vi "SQL_Delete.vi"(7 "表名":string, 8 "error in (no error)":errorcluster, 9 "值":string, 10 "列名":string, 11 "connection reference":T1) -> (0 "error out":errorcluster, 3 "connection reference 2":T1)   [LabVIEW 2018]
uses:
  <vilib>/addons/database/Connection.llb/Conn ObjectReference.ctl
  <vilib>/addons/database/Connection.llb/Conn Execute.vi
  <vilib>/addons/database/Recordset.llb/Rec Destroy - Connection.vi
  <vilib>/addons/database/NI_Database_API.lvlib
panel:
  # "语法："
  # "DELETE FROM 表名称 WHERE 列名称 = 值"
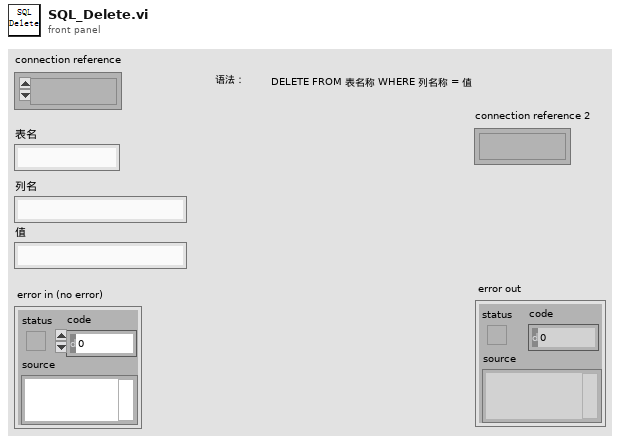
[diagram p1: front panel]
types:
  T1 = typedef "NI_Database_API.lvlib/Conn ObjectReference.ctl" = refnum<k1>
  T2 = typedef "NI_Database_API.lvlib/Rec ObjectReference.ctl" = refnum<k1>
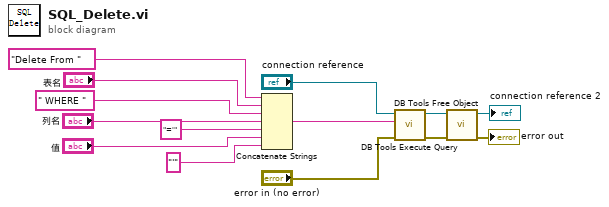
[diagram p0: block diagram]
diagram:
  n1 = Concatenate Strings("Delete From ", "表名", " WHERE " ("字符串"), "列名", "='" ("字符串"), "值", "'" ("字符串")) -> (w12:string)
  n2 = call-poly <vilib>:"DB Tools Execute Query.vi"("error in (no error)"="error in (no error)", "SQL query"=w12, "connection reference"="connection reference") -> ("error out"=w6:errorcluster, "recordset reference"=w7:T2)  [unwired: 5 in]
  n3 = call-poly <vilib>:"DB Tools Free Object.vi"("error in (no error)"=w6, "recordset reference"=w7) -> ("error out"=→"error out":errorcluster, "connection reference"=→"connection reference 2":T1)  [unwired: 8 in]
